vi "VARGLOBCOMP.vi"() -> ()   [LabVIEW 2021]
uses:
  VGLOBAL.vi
panel:
  in  "stop":bool
  in  "Boolean":bool
  out "Waveform Chart":dbl(graph)
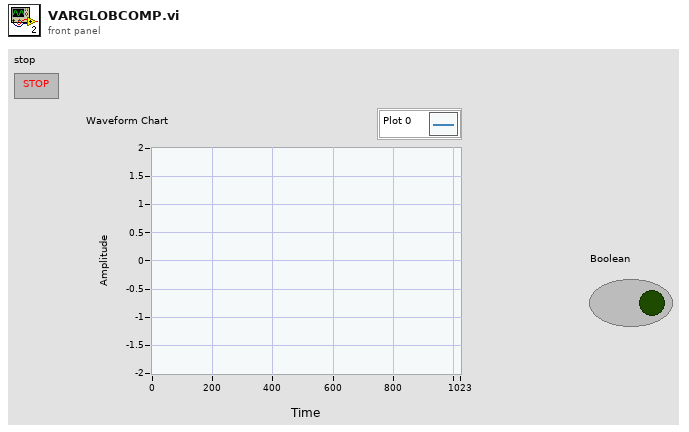
[diagram p1: front panel]
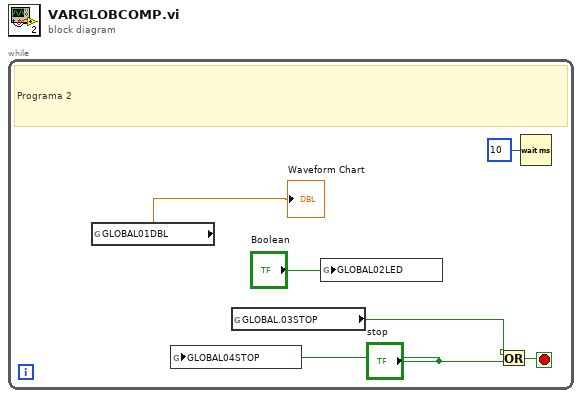
[diagram p0: block diagram]
diagram:
  n1 = while {
    stop <- w3 stop-if-true
    # "Programa 2"
    n2 = global read "VGLOBAL.vi" "GLOBAL01DBL"() -> (→"Waveform Chart":dbl)
    n3 = global write "VGLOBAL.vi" "GLOBAL04STOP"("stop") -> ()
    n4 = global read "VGLOBAL.vi" "GLOBAL.03STOP"() -> (w2:bool)
    n5 = global write "VGLOBAL.vi" "GLOBAL02LED"("Boolean") -> ()
    n6 = Or(x=w2, y="stop") -> (x .or. y?=w3:bool)
    n7 = Wait (ms)(milliseconds to wait=u32 10) -> ()  [unwired: 1 out]
  }
